vi "ZaberMoveRelative.vi"(2 "Position Indicator":refnum<vi>, 4 "Microstep resolution":dbl, 6 "distance [mm]":dbl, 8 "error in (no error)":errorcluster, 10 "Device":string, 11 "VISA Refnum in":refnum<visa-resource-name>) -> (0 "error out":errorcluster, 3 "VISA Refnum out":refnum<visa-resource-name>)   [LabVIEW 2011]
uses:
  Zaber/Zaber A Series.lvlib
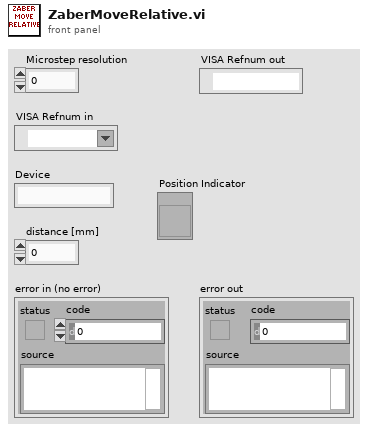
[diagram p1: front panel]
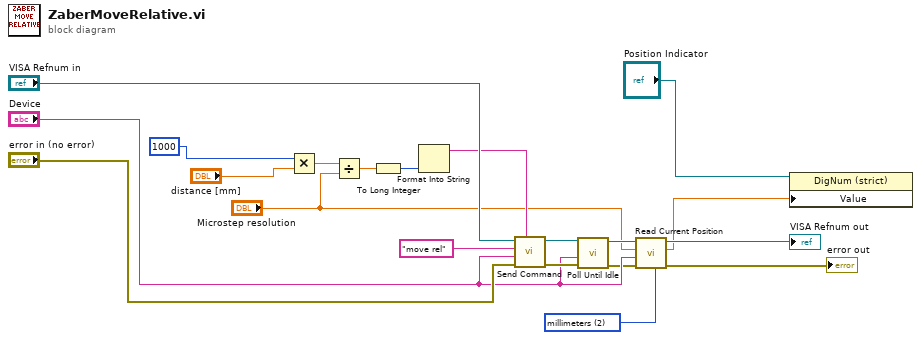
[diagram p0: block diagram]
diagram:
  w6 = u16 2 items=["microsteps", "microns", "millimeters", "inches"] ("Units (0: microsteps)")
  n1 = Multiply(x=1000, y="distance [mm]") -> (x*y=w16:dbl)
  n2 = Divide(x=w16, y="Microstep resolution") -> (x/y=w17:dbl)
  n3 = To Long Integer(number=w17) -> (32bit integer=w18:i32)
  n4 = Format Into String(w18) -> (resulting string=w19:string)  [unwired: 3 in, 1 out]
  n5 = call "Send Command.vi"("Data"=w19, "error in (no error)"="error in (no error)", "Device and Axis"="Device", "Command"="move rel", "VISA resource name"="VISA Refnum in") -> ("error out"=w10:errorcluster, "VISA resource name out"=w11:refnum<visa-resource-name>)  [unwired: 2 in, 3 out]
  n6 = call "Poll Until Idle.vi"("error in (no error)"=w10, "Device and Axis"="Device", "VISA resource name"=w11) -> ("error out"=w7:errorcluster, "VISA resource name out"=w8:refnum<visa-resource-name>)  [unwired: 7 in]
  n7 = call "Read Current Position.vi"("Units (0: microsteps)"=w6, "error in (no error)"=w7, "Device and Axis"="Device", "Microstep Size (0)"="Microstep resolution", "VISA resource name"=w8) -> ("error out"=→"error out":errorcluster, "Position"=w1:dbl, "VISA resource name out"=→"VISA Refnum out":refnum<visa-resource-name>)  [unwired: 4 in]
  n8 = property class="DigNum (strict)"(reference="Position Indicator", "Value"=w1) -> ()  [unwired: 1 in, 2 out]
